vi "getConfig.vi"(6 "Delay between send and receive [ms]":i32=100, 8 "error in (no error)":errorcluster, 11 "Monochromator in":refnum<class "Monochromator.lvclass">) -> (0 "error out":errorcluster, 1 "config-JSON string":string, 2 "config data":T1, 3 "Monochromator out":refnum<class "Monochromator.lvclass">)   [LabVIEW 2023, in "horiba.lvlib" / "Monochromator.lvclass"]
doc: "This command returns the monochromator configuration.\nPort Descriptions:\n\nlocationId Integer. Used to identify the slit location.\n1 = Front entrance (axial)\n2 = Side entrance (lateral)\n3 = Front exit (axial)\n4 = Side exit (lateral)\nslitType Integer. Used to identify the slit size.\n1 = 2mm slit\n2 = 7mm slit"
uses:
  Monochromator.lvclass
  configuration.ctl
  filterWheel.ctl
  grating.ctl
  mirror.ctl
  port.ctl
  d9b87029-586e-44ee-a6e5-d4a5e0edce38.vi
  <vilib>/JDP Science/JSONtext/Variant to JSON Text.vi
  <vilib>/JDP Science/JSONtext/Set Item.vi
  <vilib>/JDP Science/JSONtext/LVClass Serializer/JSONtext LVClass Serializer.lvclass
  GenericDevice/GenericDevice.lvclass
  <vilib>/JDP Science/JSONtext/JSONtext.lvlib
panel:
  # "Connector Pane"
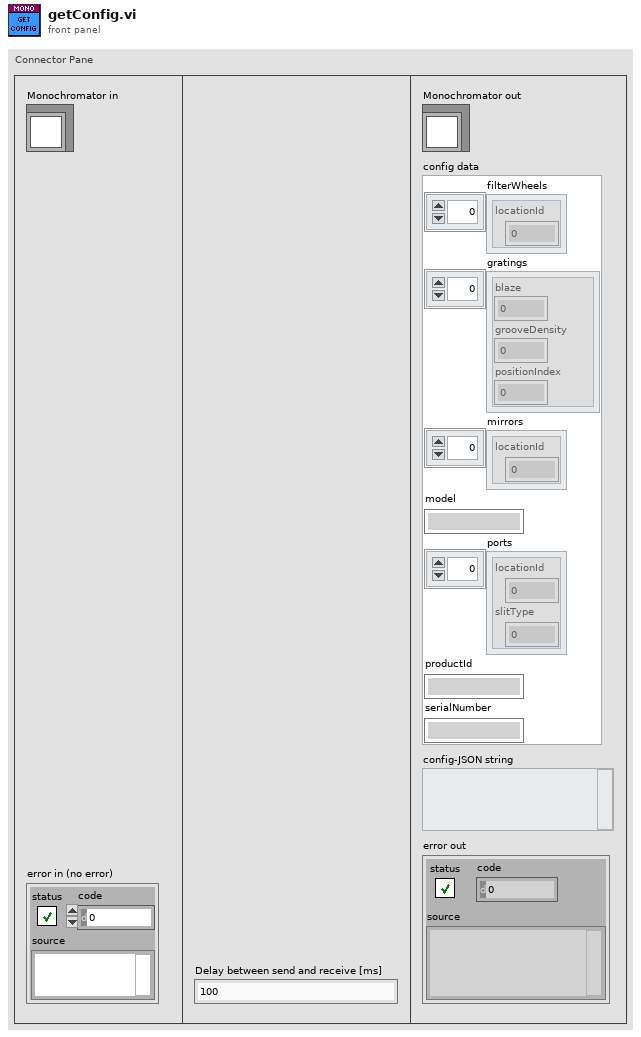
[diagram p1: front panel]
types:
  T1 = typedef "horiba.lvlib/Monochromator.lvclass/configuration.ctl" = cluster{"filterWheels":T2[], "gratings":T3[], "mirrors":T4[], "model":string, "ports":T5[], "productId":string, "serialNumber":string}
  T2 = typedef "horiba.lvlib/Monochromator.lvclass/filterWheel.ctl" = cluster{"locationId":i32}
  T3 = typedef "horiba.lvlib/Monochromator.lvclass/grating.ctl" = cluster{"blaze":i32, "grooveDensity":i32, "positionIndex":i32}
  T4 = typedef "horiba.lvlib/Monochromator.lvclass/mirror.ctl" = cluster{"locationId":i32}
  T5 = typedef "horiba.lvlib/Monochromator.lvclass/port.ctl" = cluster{"locationId":i32, "slitType":i32}
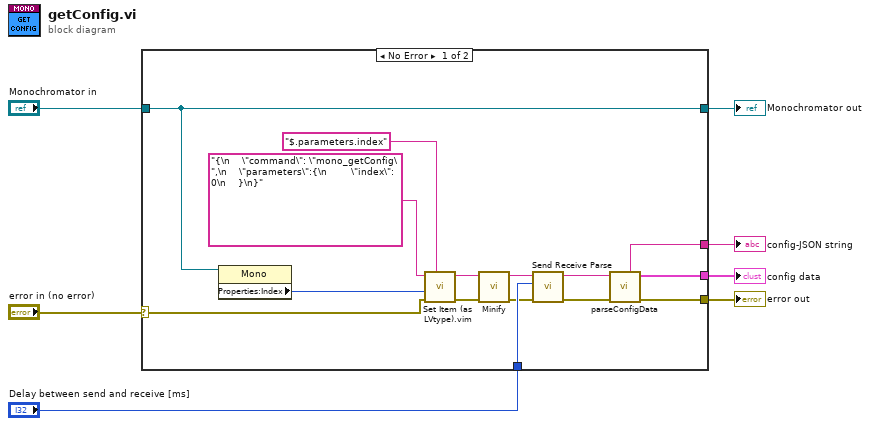
[diagram p0: block diagram]
diagram:
  n1 = case shown="No Error" "error in (no error)" {
    selector: "error in (no error)" -> [w17 w23]
    tunnel: [w9 w23] -> w6
    tunnel: [w19 w22] -> w4
    tunnel: "Monochromator in" -> [w19 w22]
    tunnel: "Delay between send and receive [ms]" -> [w15 _]
    tunnel: [w11 _] -> w2
    tunnel: [w8 _] -> w1
    frame No Error {
      n2 = property class="Mono"(reference=w19) -> ("Properties:Index"=w18:i32)  [unwired: 1 in, 2 out]
      n3 = call "Set Item (as LVtype).vim"("$Path or Item Name"="$.parameters.index", "error in (no error)"=w17, "Anything"=w18, "JSON"="{\n    \"command\": \"mono_getConfig\",\n    \"parameters\":{\n        \"index\": 0\n    }\n}") -> ("error out"=w16:errorcluster, "<JSON>"=w13:string)  [unwired: 4 in, 1 out]
      n4 = call <vilib>:"Minify.vi"("error in (no error)"=w16, "JSON"=w13) -> ("error out"=w14:errorcluster, "<JSON>"=w12:string)  [unwired: 7 in, 1 out]
      n5 = call "Send Receive Parse.vi"("error in"=w14, "Delay between send and receive [ms]"=w15, "<JSON>"=w12) -> ("error out"=w10:errorcluster, "results-JSON string"=w11:string)  [unwired: 6 in, 1 out]
      n6 = call "parseConfigData.vi"("error in (no error)"=w10, "results-JSON string"=w11) -> ("error out"=w9:errorcluster, "config data"=w8:T1)  [unwired: 6 in, 2 out]
    }
    frame Error {
    }
  }
  "error out" <- w6
  "Monochromator out" <- w4
  "config-JSON string" <- w2
  "config data" <- w1
